vi "CRYLimit Table Offset.vi"(0 "Limit in":cluster{"Numeric":dbl, "Numeric 2":dbl}[](array[cluster]) {"Numeric 2" format="%.2f"; "Numeric" format="%.2f"}, 1 "Data unit":string, 5 "X offset":dbl format="%.2f", 7 "Y offset":dbl format="%.2f", 9 "Starting Column":i32, 11 "Number of columns":i32, 12 "x Unit":u16(ring) items=["dB", "%"], 13 "y Unit":u16(ring) items=["dB", "%"]) -> (4 "Limit out":cluster{"Numeric":dbl, "Log Out":dbl}[](array[cluster]))   [LabVIEW 2013]
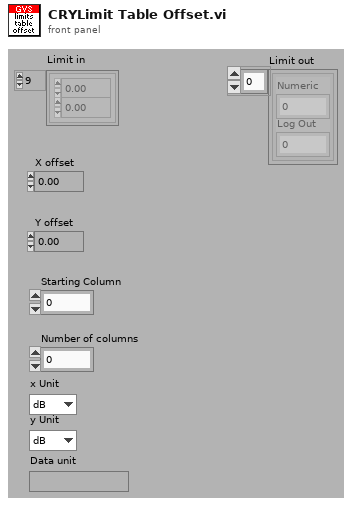
[diagram p1: front panel]
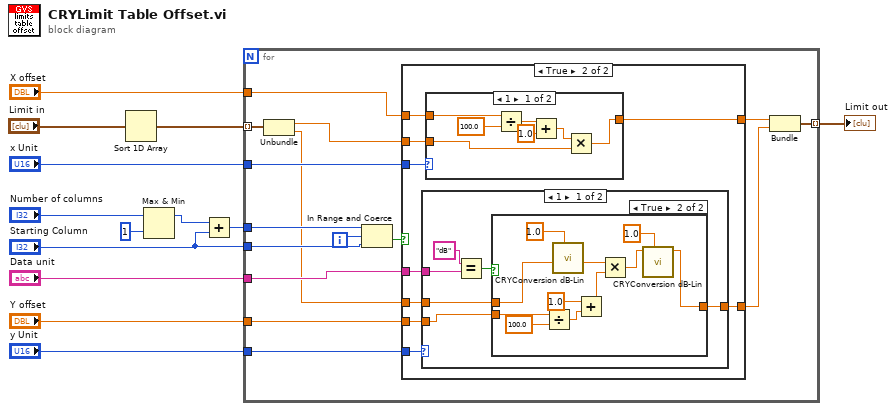
[diagram p0: block diagram]
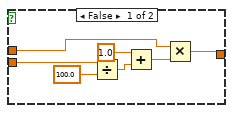
[diagram p3: hidden frame]
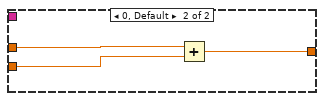
[diagram p4: hidden frame]
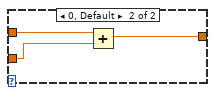
[diagram p5: hidden frame]
diagram:
  n1 = Sort 1D Array(array="Limit in") -> (sorted array=w1:cluster{"Numeric":dbl, "Numeric 2":dbl}[])
  n2 = Max & Min(x="Number of columns", y=1 ("Number of columns")) -> (max(x,y)=w11:i32)  [unwired: 1 out]
  n3 = Add(x=w11, y="Starting Column") -> (x+y=w10:i32)
  n4 = for {
    tunnel: "Y offset" -> [w28]
    tunnel: "Starting Column" -> [w25]
    tunnel: w10 -> [w24]
    tunnel: "X offset" -> [w23]
    tunnel: "x Unit" -> [w22]
    tunnel: "y Unit" -> [w21]
    tunnel: "Data unit" -> [w20]
    tunnel: w1 -> [w19] mode=indexing
    tunnel: [w14] -> w2 mode=indexing
    i -> [w26]
    n5 = Unbundle(w19) -> ("Numeric"=w18:dbl, "Numeric 2"=w17:dbl)
    n6 = In Range and Coerce(upper limit=w24, x=w26, lower limit=w25) -> (In Range?=w27:bool)  [unwired: 1 out]
    n7 = case shown="True" w27 {
      tunnel: w28 -> [_ w39]
      tunnel: w17 -> [w30 w38]
      tunnel: [w30 w37] -> w15
      tunnel: w18 -> [w29 w36]
      tunnel: [w29 w35] -> w16
      tunnel: w23 -> [_ w34]
      tunnel: w22 -> [_ w33]
      tunnel: w21 -> [_ w32]
      tunnel: w20 -> [_ w31]
      frame False {
      }
      frame True {
        n8 = case shown="1" w32 {
          tunnel: w39 -> [w42 w66]
          tunnel: w38 -> [w41 w65]
          tunnel: [w40 w64] -> w37
          tunnel: w31 -> [w45 _]
          frame 1 {
            n9 = Equal?(x="dB", y=w45) -> (x = y?=w43:bool)
            n10 = case shown="True" w43 {
              tunnel: w42 -> [w52 w58]
              tunnel: w41 -> [w47 w56]
              tunnel: [w46 w55] -> w40
              frame False {
                n11 = Divide(x=w52, y=100.0) -> (x/y=w50:dbl)
                n12 = Add(x=1.0, y=w50) -> (x+y=w48:dbl)
                n13 = Multiply(x=w47, y=w48) -> (x*y=w46:dbl)
              }
              frame True {
                n14 = Divide(x=w58, y=100.0) -> (x/y=w61:dbl)
                n15 = call "CRYConversion dB-Lin.vi"("dB ref."=1.0, "Log In"=w56) -> ("Lin Out"=w59:dbl)  [unwired: 4 in, 3 out]
                n16 = Add(x=1.0, y=w61) -> (x+y=w63:dbl)
                n17 = Multiply(x=w59, y=w63) -> (x*y=w60:dbl)
                n18 = call "CRYConversion dB-Lin.vi"("dB ref."=1.0, "Lin In"=w60) -> ("Log Out"=w55:dbl)  [unwired: 4 in, 3 out]
              }
            }
          }
          frame 0, Default {
            n19 = Add(x=w65, y=w66) -> (x+y=w64:dbl)
          }
        }
        n20 = case shown="1" w33 {
          tunnel: w36 -> [w68 w76]
          tunnel: [w67 w75] -> w35
          tunnel: w34 -> [w73 w74]
          frame 1 {
            n21 = Divide(x=w73, y=100.0) -> (x/y=w71:dbl)
            n22 = Add(x=w71, y=1.0) -> (x+y=w69:dbl)
            n23 = Multiply(x=w69, y=w68) -> (x*y=w67:dbl)
          }
          frame 0, Default {
            n24 = Add(x=w74, y=w76) -> (x+y=w75:dbl)
          }
        }
      }
    }
    n25 = Bundle("Numeric"=w16, "Log Out"=w15) -> (w14:cluster{"Numeric":dbl, "Log Out":dbl})  [unwired: 1 out]
  }
  "Limit out" <- w2
